vi "Append Waveform.vi"(8 "Error":errorcluster, 9 "Waveform To Append":T1, 11 "WavBuf":refnum<class "WavBuf.lvclass">) -> (0 "Error Out":errorcluster, 3 "WavBuf Out":refnum<class "WavBuf.lvclass">, 5 "Tf Out":timestamp)   [LabVIEW 2020, in "WavBuf.lvclass"]
uses:
  WavBuf.lvclass
  Universal Controls/Waveform_Data.ctl
  WavBuf.lvclass/WavBuf.ctl
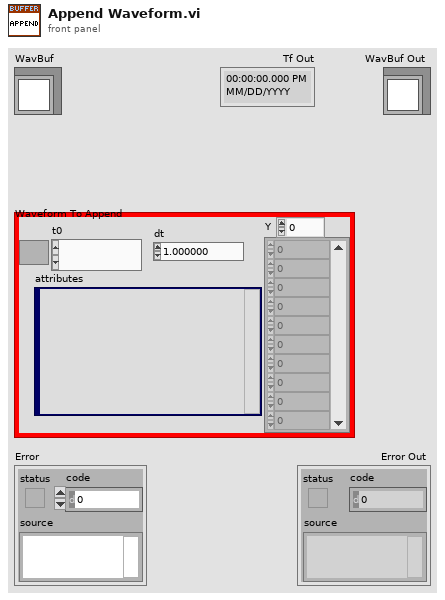
[diagram p1: front panel]
types:
  T1 = typedef "Waveform_Data.ctl" = waveform(dbl)
  T2 = typedef "Ref_DVR_Buffer.ctl" = refnum<data-value>
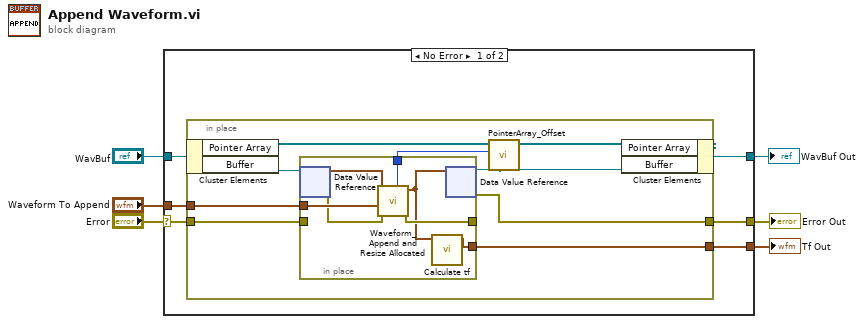
[diagram p0: block diagram]
diagram:
  n1 = case shown="No Error" "Error" {
    selector: "Error" -> [w10 w30]
    tunnel: [w8 w30] -> w5
    tunnel: [w12 w29] -> w3
    tunnel: "WavBuf" -> [w11 w29]
    tunnel: "Waveform To Append" -> [w9 _]
    tunnel: [w7 _] -> w1
    frame No Error {
      n2 = in-place {
        in-place-border: w10 -> [w21]
        in-place-border: [w14] -> w8
        in-place-border: w9 -> [w20]
        in-place-border: [w13] -> w7
        n3 = in-place-cluster #1(w11) -> ("Pointer Array"=w16:refnum<class "_Pointer.lvclass">[], "Buffer"=w19:T2)
        n4 = in-place {
          in-place-border: w21 -> [_]
          in-place-border: [w24] -> _
          in-place-border: [w28] -> w17
          in-place-border: w20 -> [w26]
          in-place-border: [w22] -> w13
          n5 = in-place-dvr #2(w19) -> (w27:T1, w25:errorcluster)
          n6 = call "Waveform_Append and Resize Allocated.vi"("Error"=w25, "Append"=w26, "Waveform"=w27) -> ("Error Out"=w24:errorcluster, "Waveform Out"=w23:T1, "Offset Out"=w28:i32)  [unwired: 6 in]
          n7 = call "Calculate tf.vi"("Waveform"=w23) -> ("Tf Out"=w22:timestamp)  [unwired: 10 in]
          n8 = in-place-dvr #2(w23) -> (w18:T2, w14:errorcluster)
        }
        n9 = call "PointerArray_Offset.vi"("Buffer"=w18, "Total Starting Offset"=w17, "Pointer Array"=w16) -> ("Pointer Array Out"=w15:refnum<class "_Pointer.lvclass">[])  [unwired: 8 in]
        n10 = in-place-cluster #1("Pointer Array"=w15, "Buffer"=w18) -> (w12:refnum<class "WavBuf.lvclass">)
      }
    }
    frame Error {
    }
  }
  "Error Out" <- w5
  "WavBuf Out" <- w3
  "Tf Out" <- w1
